vi "Update Element.vi"(8 "g":dbl, 9 "f":dbl, 10 "index":i32, 11 "Priority Queue in":refnum<class "NI_Robotics_Priority Queue.lvclass">) -> (3 "Priority Queue out":refnum<class "NI_Robotics_Priority Queue.lvclass">)   [LabVIEW 2017, in "NI_Robotics_Priority Queue.lvclass"]
uses:
  <vilib>/robotics/Navigation/shared/Priority Queue/NI_Robotics_Priority Queue.lvclass
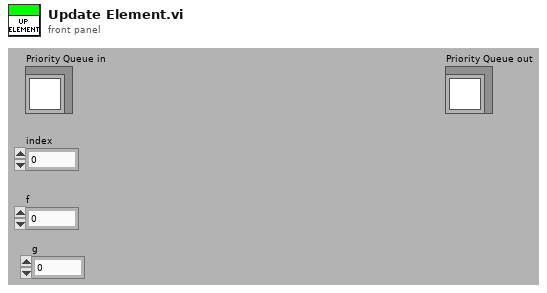
[diagram p1: front panel]
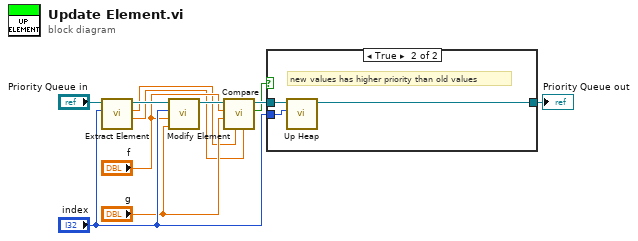
[diagram p0: block diagram]
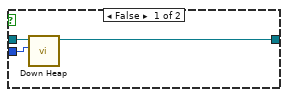
[diagram p2: hidden frame]
diagram:
  n1 = call <vilib>:"Extract Element.vi"("index"="index", "Priority Queue in"="Priority Queue in") -> ("g"=w1:dbl, "f"=w2:dbl, "Priority Queue out"=w10:refnum<class "NI_Robotics_Priority Queue.lvclass">)  [unwired: 6 in, 1 out]
  n2 = call <vilib>:"Modify Element.vi"("g"="g", "f"="f", "index"="index", "Priority Queue in"=w10) -> ("Priority Queue out"=w7:refnum<class "NI_Robotics_Priority Queue.lvclass">)  [unwired: 7 in]
  n3 = call <vilib>:"Compare.vi"("gB"=w1, "fB"=w2, "gA"="g", "fA"="f", "Priority Queue in"=w7) -> ("priority(A) > priority(B)"=w5:bool, "Priority Queue out"=w6:refnum<class "NI_Robotics_Priority Queue.lvclass">)  [unwired: 5 in]
  n4 = case shown="True" w5 {
    tunnel: w6 -> [w14 w17]
    tunnel: "index" -> [w13 w16]
    tunnel: [w12 w15] -> w8
    frame False {
      n5 = call <vilib>:"Down Heap.vi"("index"=w13, "Astar Open List in"=w14) -> ("Astar Open List out"=w12:refnum<class "NI_Robotics_Priority Queue.lvclass">)  [unwired: 8 in, 1 out]
    }
    frame True {
      # "new values has higher priority than old values"
      n6 = call <vilib>:"Up Heap.vi"("index"=w16, "Astar Open List in"=w17) -> ("Astar Open List out"=w15:refnum<class "NI_Robotics_Priority Queue.lvclass">)  [unwired: 8 in, 1 out]
    }
  }
  "Priority Queue out" <- w8
